vi "CLI Demo.vi"() -> ()   [LabVIEW 2020]
uses:
  Basic Example/Dummy/Dummy.lvclass
panel:
  out "error out":errorcluster
  in  "Report type":enum32{"txt", "xml"}(radio)
  out "standard output":string
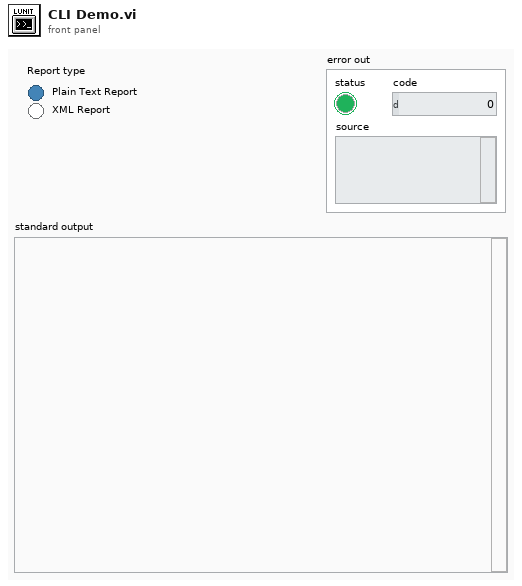
[diagram p1: front panel]
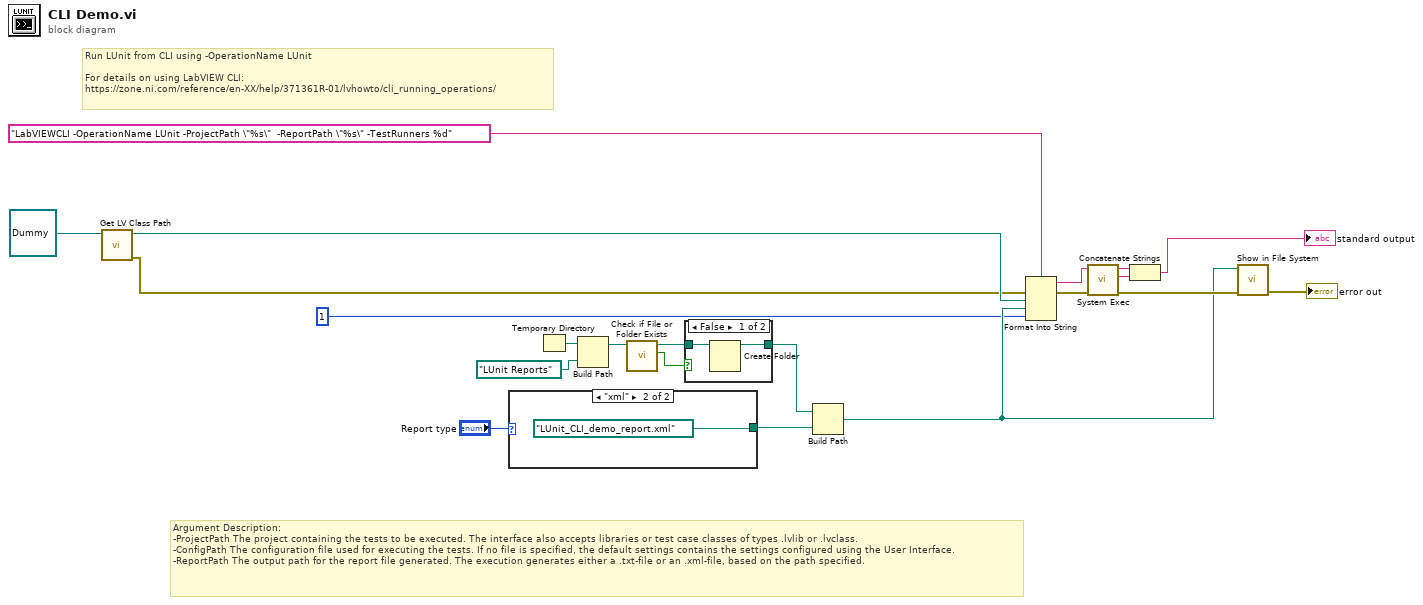
[diagram p0: block diagram]
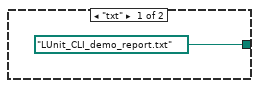
[diagram p3: hidden frame]
diagram:
  # "Run LUnit from CLI using -OperationName LUnit\n\nFor details on using LabVIEW CLI:\nhttps://zone.ni.com/reference/en-XX/help/371361R-01/lvhowto/cli_running_operations/"
  # "Argument\tDescription:\n-ProjectPath\tThe project containing the tests to be executed. The interface also accepts libraries or test case classes of types .lvlib or .lvclass. \n-ConfigPath\tThe configuration file used for executing the tests. If no file is specified, the default settings contains the settings configured using the User Interface.\n-ReportPath\tThe output path for the report file generated. The execution generates either a .txt-file or an .xml-file, based on the path specified."
  n1 = call <vilib>:"Get LV Class Path.vi"("object"=refnum<class "Dummy.lvclass"> refnum ("Dummy.lvclass")) -> ("error out"=w13:errorcluster, "class path"=w19:path)  [unwired: 9 in]
  n2 = case shown="\"xml\"" "Report type" {
    tunnel: [path "LUnit_CLI_demo_report.txt" ("name or relative path") path "LUnit_CLI_demo_report.xml" ("name or relative path")] -> w14
    frame "txt" {
    }
    frame "xml" {
    }
  }
  n3 = Temporary Directory() -> (w9:path)
  n4 = Build Path(base path=w9, name or relative path=path "LUnit Reports") -> (appended path=w10:path)
  n5 = call <vilib>:"Check if File or Folder Exists.vi"("path"=w10) -> ("file or folder exists?"=w1:bool, "dup path"=w3:path)  [unwired: 8 in, 1 out]
  n6 = case shown="False" w1 {
    tunnel: w3 -> [w25 w26]
    tunnel: [w24 w26] -> w2
    frame False {
      n7 = Create Folder(path (use dialog)=w25) -> (created path=w24:path)  [unwired: 2 in, 2 out]
    }
    frame True {
    }
  }
  n8 = Build Path(base path=w2, name or relative path=w14) -> (appended path=w7:path)
  n9 = Format Into String(format string="LabVIEWCLI -OperationName LUnit -ProjectPath \"%s\"  -ReportPath \"%s\" -TestRunners %d", error in=w13, w19, w7, 1 ("input 3")) -> (resulting string=w11:string, error out=w18:errorcluster)  [unwired: 1 in]
  n10 = call <vilib>:"System Exec.vi"("error in (no error)"=w18, "command line"=w11) -> ("error out"=w17:errorcluster, "standard error"=w4:string, "standard output"=w16:string)  [unwired: 6 in, 1 out]
  n11 = Concatenate Strings(w16, w4) -> (→"standard output":string)
  n12 = call <vilib>:"Show in File System.vi"("error in (no error)"=w17, "file or directory path"=w7) -> ("error out"=→"error out":errorcluster)  [unwired: 9 in]
